vi "configuration.vi"(4 "force_read?":bool, 6 "custom_file":path, 7 "command":T1=enum."read_config", 8 "error in (no error)":errorcluster, 10 "project_file":path, 11 "config in":T2) -> (0 "error out":errorcluster, 3 "config out":T2)   [LabVIEW 2015, in "lv-builder.lvlib"]
doc: "This VI is able to read/write configuration from all the associated modules defined in the master data cluster. It also acts as a functional global/data store in the event that no data has changed since the last write. It will self-initialize and well set an internal flag in the event an error is encountered when reading. If no command is provided, it will default to the read command."
uses:
  lv-builder.lvlib
  public/_controls/configuration.ctl
  _controls/command_configuration.ctl
  lv-build/lv-build.lvlib
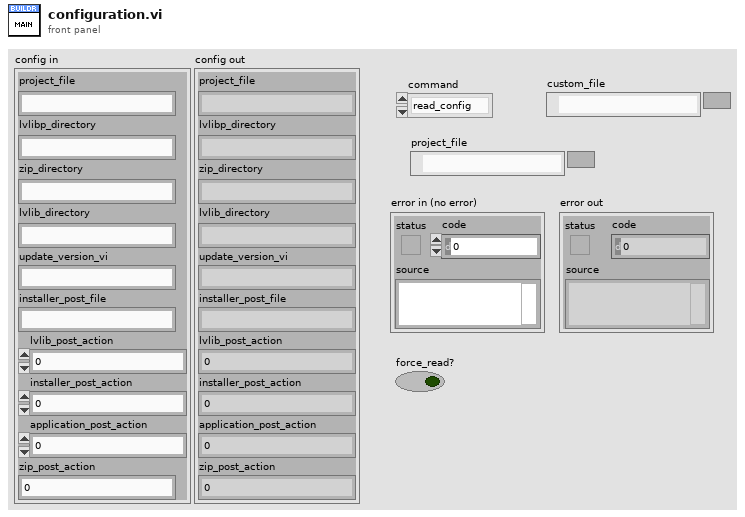
[diagram p1: front panel]
types:
  T1 = typedef "lv-builder.lvlib/command_configuration.ctl" = enum16{"<config_command>", "read_config", "write_config", "<null>"}
  T2 = typedef "lv-builder.lvlib/configuration.ctl" = cluster{"project_file":string, "lvlibp_directory":string, "zip_directory":string, "lvlib_directory":string, "update_version_vi":string, "installer_post_file":string, "lvlib_post_action":u16, "installer_post_action":u16, "application_post_action":u16, "zip_post_action":u16}
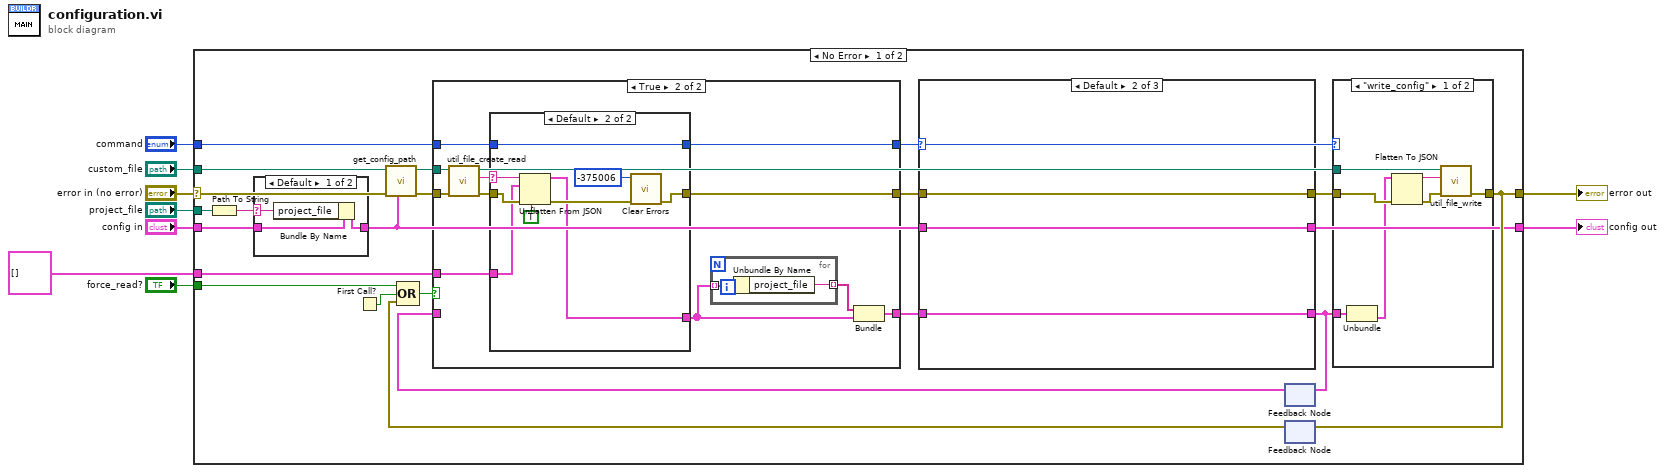
[diagram p0: block diagram]
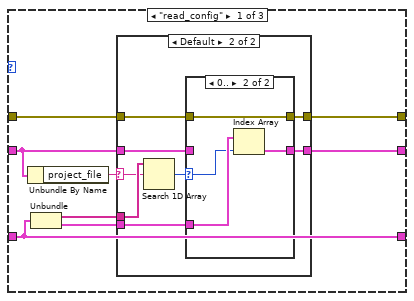
[diagram p2: hidden frame]
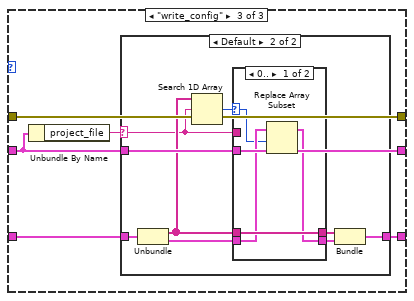
[diagram p5: hidden frame]
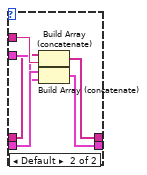
[diagram p7: hidden frame]
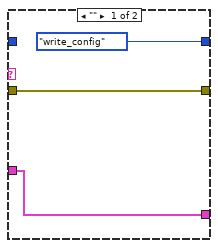
[diagram p9: hidden frame]
diagram:
  n1 = case shown="No Error" "error in (no error)" {
    selector: "error in (no error)" -> [w12 w124]
    tunnel: "command" -> [w24 _]
    tunnel: [w31 w124] -> w5
    tunnel: "config in" -> [w15 _]
    tunnel: "custom_file" -> [w14 _]
    tunnel: [w22 _] -> w4
    tunnel: "force_read?" -> [w28 _]
    tunnel: T2[] [] ("default") -> [w25 _]
    tunnel: "project_file" -> [w17 _]
    frame No Error {
      n2 = Path To String(path=w17) -> (string=w16:string)
      n3 = case shown="Default" w16 {
        selector: w16 -> [w120 _]
        tunnel: w15 -> [w122 w123]
        tunnel: [w121 w123] -> w10
        frame Default {
          n4 = Bundle By Name(cluster=w122, "project_file"=w120) -> (w121:T2)
        }
        frame "" {
        }
      }
      n5 = First Call?() -> (First Call?: T/F=w29:bool)
      n6 = call "get_config_path.vi"("configuration"=w10, "error in (no error)"=w12, "custom_path"=w14) -> ("error out"=w11:errorcluster, "lv_build_config_path"=w13:path)  [unwired: 7 in]
      n7 = feedback #1() -> (w26:cluster{string[], "default":T2[]})  [unwired: 1 in]
      n8 = feedback #2() -> (w30:errorcluster)  [unwired: 1 in]
      n9 = Compound Arithmetic op=OR(w28, w29, w30) -> (w27:bool)
      n10 = case shown="True" w27 {
        tunnel: w26 -> [w86 _]
        tunnel: w11 -> [w85 w95]
        tunnel: w13 -> [_ w96]
        tunnel: [w85 w93] -> w20
        tunnel: w25 -> [_ w97]
        tunnel: w24 -> [w84 w92]
        tunnel: [w84 w91] -> w21
        tunnel: [w86 w89] -> w23
        frame False {
        }
        frame True {
          n11 = call "util_file_create_read.vi"("error in (no error)"=w95, "config_path"=w96) -> ("error out"=w94:errorcluster, "string"=w90:string)  [unwired: 8 in]
          n12 = case shown="Default" w90 {
            selector: w90 -> [_ w107]
            tunnel: w97 -> [w101 w109]
            tunnel: [w101 w108] -> w88
            tunnel: w94 -> [w102 w111]
            tunnel: [w102 w103] -> w93
            tunnel: w92 -> [_ w106]
            tunnel: [command_configuration."write_config" ("command") w106] -> w91
            frame "" {
            }
            frame Default {
              n13 = Unflatten From JSON(JSON string=w107, type and defaults=w109, default null elements? (F)=TRUE, error in (no error)=w111) -> (value=w108:T2[], error out=w110:errorcluster)  [unwired: 3 in]
              n14 = call <vilib>:"Clear Errors.vi"("error in (no error)"=w110, "specific error code to clear (0: all)"=-375006) -> ("error out"=w103:errorcluster)  [unwired: 4 in, 1 out]
            }
          }
          n15 = for {
            tunnel: w88 -> [w99] mode=indexing
            tunnel: [w98] -> w87 mode=indexing
            n16 = Unbundle By Name(w99) -> ("project_file"=w98:string)
          }
          n17 = Bundle(w87, "default"=w88) -> (w89:cluster{string[], "default":T2[]})  [unwired: 1 in]
        }
      }
      n18 = case shown="Default" w21 {
        tunnel: w10 -> [w32 w57 w59]
        tunnel: [w39 w56 w62] -> w18
        tunnel: w23 -> [w39 w56 w60]
        tunnel: [w35 w57 w59] -> w22
        tunnel: w20 -> [w34 w55 w58]
        tunnel: [w33 w55 w58] -> w19
        frame "read_config" {
          n19 = Unbundle By Name(w32) -> ("project_file"=w36:string)
          n20 = Unbundle(w39) -> (w38:string[], "default"=w37:T2[])
          n21 = case shown="Default" w36 {
            selector: w36 -> [_ w45]
            tunnel: w38 -> [_ w48]
            tunnel: w37 -> [_ w47]
            tunnel: [_ w44] -> w35
            tunnel: w34 -> [w40 w43]
            tunnel: [w40 w42] -> w33
            tunnel: w32 -> [_ w41]
            frame "" {
            }
            frame Default {
              n22 = Search 1D Array(1D array=w48, element=w45) -> (index of element=w46:i32)  [unwired: 1 in]
              n23 = case shown="0.." w46 {
                selector: w46 -> [_ w53]
                tunnel: w47 -> [_ w54]
                tunnel: [w49 w52] -> w44
                tunnel: w43 -> [w50 w51]
                tunnel: [w50 w51] -> w42
                tunnel: w41 -> [w49 _]
                frame Default {
                }
                frame 0.. {
                  n24 = Index Array(array=w54, index=w53) -> (element=w52:T2)
                }
              }
            }
          }
        }
        frame Default {
        }
        frame "write_config" {
          n25 = Unbundle By Name(w59) -> ("project_file"=w61:string)
          n26 = case shown="Default" w61 {
            selector: w61 -> [_ w64]
            tunnel: [w63 w70] -> w62
            tunnel: w59 -> [_ w68]
            tunnel: w60 -> [w63 w66]
            frame "" {
            }
            frame Default {
              n27 = Unbundle(w66) -> (w65:string[], "default"=w67:T2[])
              n28 = Search 1D Array(1D array=w65, element=w64) -> (index of element=w72:i32)  [unwired: 1 in]
              n29 = case shown="0.." w72 {
                selector: w72 -> [w73 _]
                tunnel: w67 -> [w76 w82]
                tunnel: [w75 w80] -> w71
                tunnel: w65 -> [w77 w78]
                tunnel: [w77 w79] -> w69
                tunnel: w68 -> [w74 w81]
                tunnel: w64 -> [_ w83]
                frame 0.. {
                  n30 = Replace Array Subset(array=w76, new element=w74, index=w73) -> (w75:T2[])
                }
                frame Default {
                  n31 = Build Array (concatenate)(w78, w83) -> (w79:string[])
                  n32 = Build Array (concatenate)(w82, w81) -> (w80:T2[])
                }
              }
              n33 = Bundle(w69, "default"=w71) -> (w70:cluster{string[], "default":T2[]})  [unwired: 1 in]
            }
          }
        }
      }
      n34 = feedback-in #1(w18) -> ()
      n35 = case shown="\"write_config\"" w21 {
        tunnel: w18 -> [w115 _]
        tunnel: w19 -> [w116 w119]
        tunnel: [w113 w119] -> w31
        tunnel: w13 -> [w114 _]
        frame "write_config" {
          n36 = Unbundle(w115) -> ("default"=w112:T2[])  [unwired: 1 out]
          n37 = Flatten To JSON(anything=w112, error in (no error)=w116) -> (JSON string=w118:string, 11:w117:errorcluster)  [unwired: 1 in]
          n38 = call "util_file_write.vi"("error in (no error)"=w117, "string"=w118, "config_path"=w114) -> ("error out"=w113:errorcluster)  [unwired: 8 in]
        }
        frame Default {
        }
      }
      n39 = feedback-in #2(w31) -> ()
    }
    frame Error {
      # "If an error is wired in, be sure to skip over functionality to preserve the original error"
    }
  }
  "config out" <- w4
  "error out" <- w5
